vi "IMAQ Gerchberg Iteration.vi"(0 "field":T2, 1 "Original Source":dbl[][](array[numeric]), 2 "n_grid":i32=300, 3 "forward distance":dbl=0.02, 4 "Original Target":dbl[][](array[numeric]), 5 "error in (no error)":errorcluster, 6 "Source":T1, 7 "Target":T1, 8 "Source Phase":T1, 9 "Target Phase":T1) -> (10 "Source Intensity":dbl[][](array[numeric]), 11 "Target Intensity":dbl[][](array[numeric]), 12 "Source Phase":dbl[][](array[numeric]), 13 "Target Phase":dbl[][](array[numeric]), 14 "field out":T2, 15 "Target Intensity\n RMS Error":dbl(graph)=285.2404780234725, 19 "error out":errorcluster)   [LabVIEW 2012, in "LightPipes.lvlib"]
uses:
  LightPipes.lvlib
  <vilib>/vision/Image Controls.llb/IMAQ Image.ctl
panel:
  out "Source Phase":T1(plugin-control)
  out "Target Phase":T1(plugin-control)
  out "Source":T1(plugin-control)
  out "Target":T1(plugin-control)
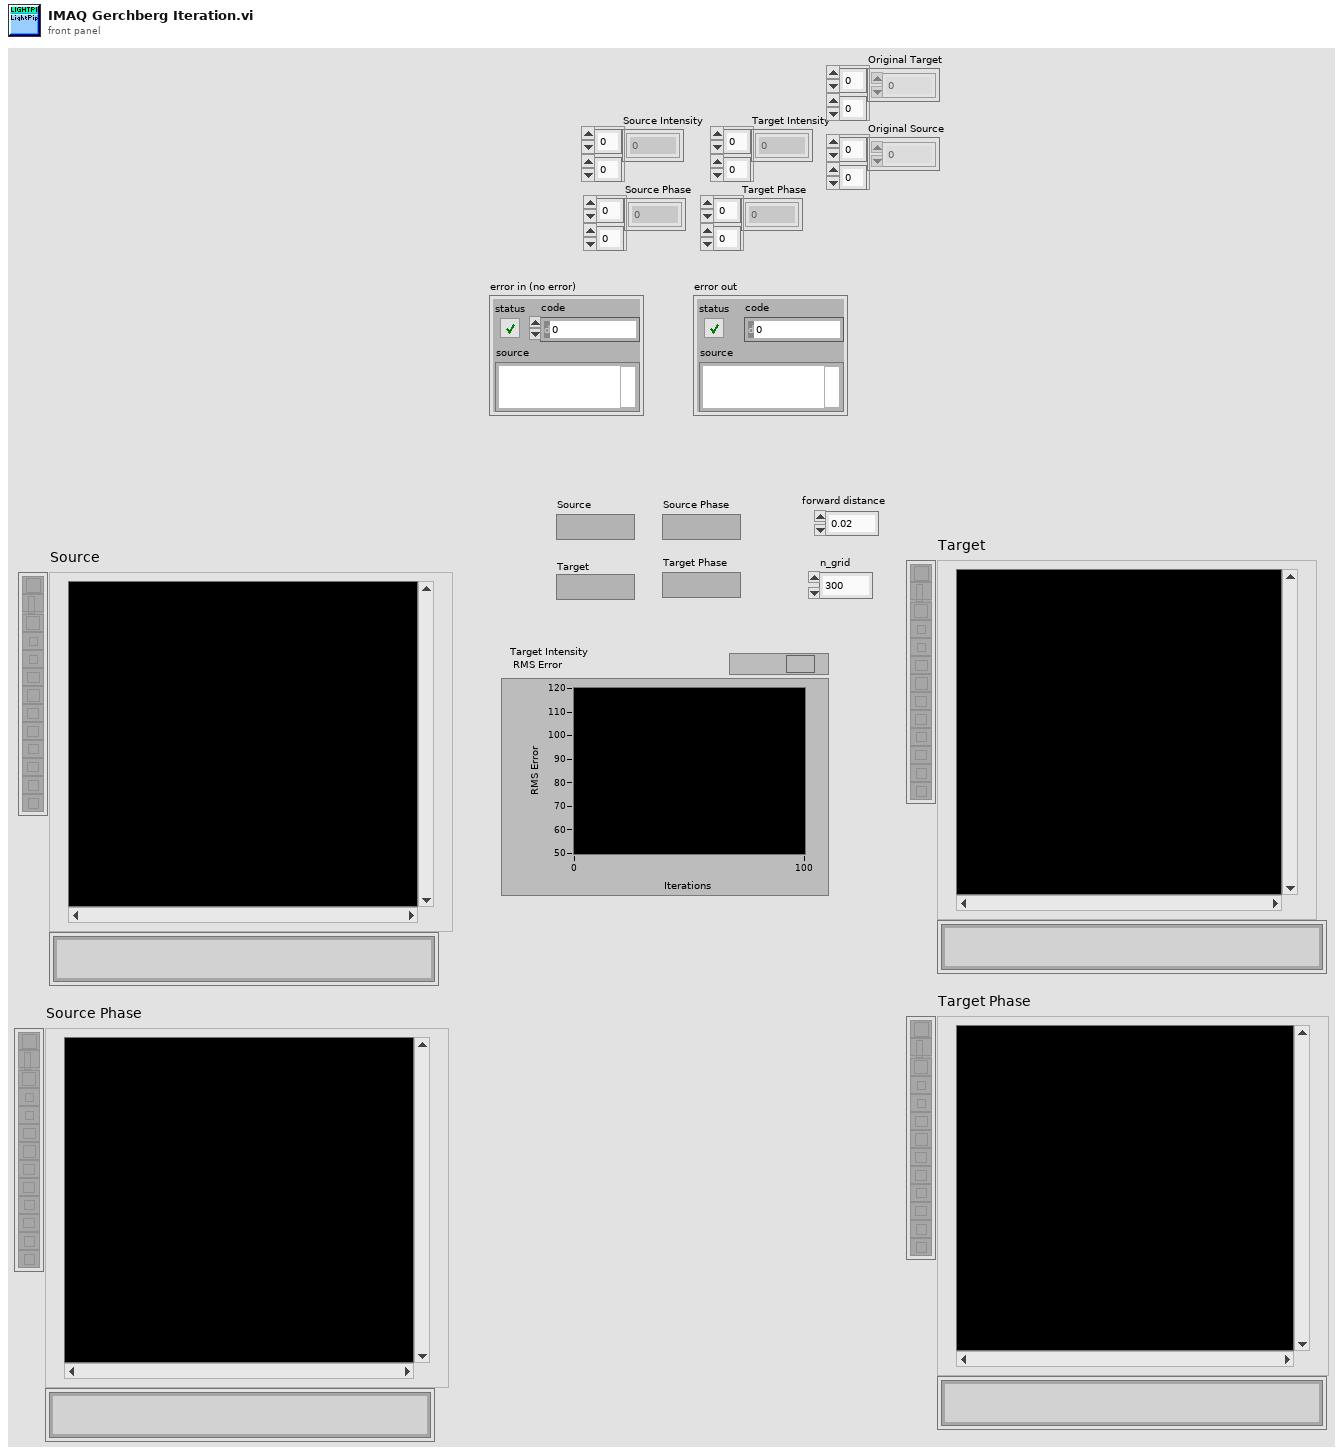
[diagram p1: front panel]
types:
  T1 = typedef "IMAQ Image.ctl" = refnum<image>
  T2 = cluster{"n_grid":i32, "@dummy control@":i8, "@dummy control@":i8, "@dummy control@":i8, "@dummy control@":i8, "size":dbl, "lambda":dbl, "int1":i32, "int2":i32, "int3":i32, "@dummy control@":i8, "@dummy control@":i8, "@dummy control@":i8, "@dummy control@":i8, "double1":dbl, "double2":dbl, "double3":dbl, "real":u32, "imaginary":u32}
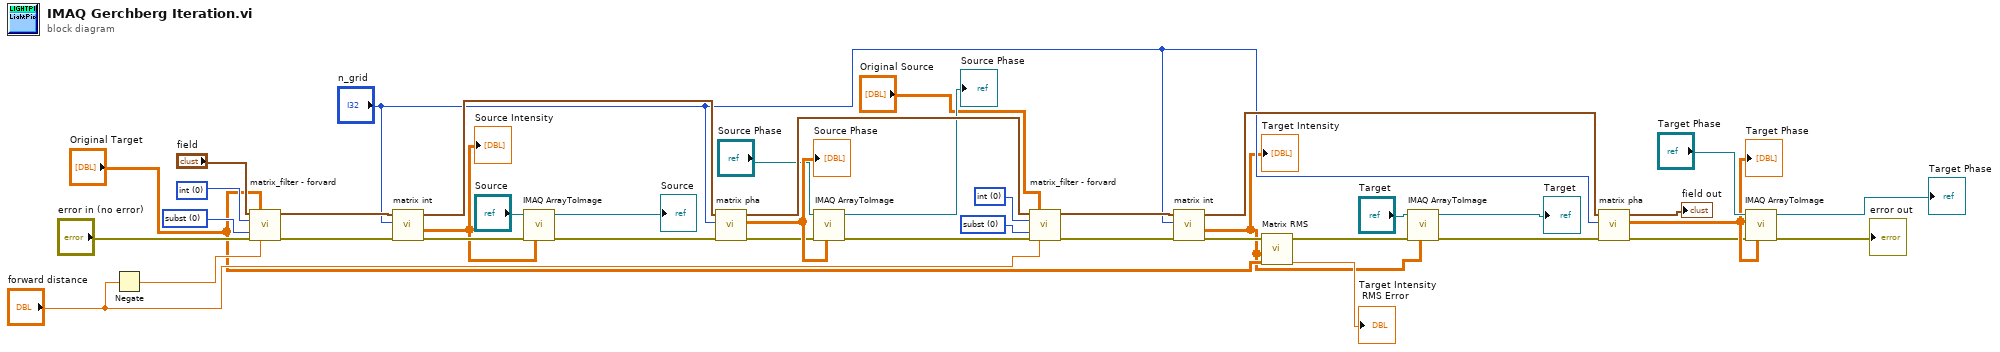
[diagram p0: block diagram]
diagram:
  w36 = i16 0 items=["int", "pha"] ("intensity/phase")
  w37 = i16 0 items=["subst", "mult"] ("multiplication/substitution")
  w38 = i16 0 items=["int", "pha"] ("intensity/phase")
  w39 = i16 0 items=["subst", "mult"] ("multiplication/substitution")
  n1 = Negate(x="forward distance") -> (-x=w35:dbl)
  n2 = call "matrix_filter - forvard.vi"("field"="field", "matrix in"="Original Target", "intensity/phase"=w36, "multiplication/substitution"=w37, "error in (no error)"="error in (no error)", "forward distance"=w35) -> ("field out"=w32:T2, "error out"=w23:errorcluster)  [unwired: 8 in]
  n3 = call "matrix int.vi"("error in (no error)"=w23, "n_grid"="n_grid", "field"=w32) -> ("error out"=w22:errorcluster, "matrix out 2D"=w3:dbl[][], "field out"=w31:T2)  [unwired: 6 in]
  "Source Intensity" <- w3
  n4 = call "IMAQ ArrayToImage"("Image Pixels (Float)"=w3, "error in (no error)"=w22, "Image"="Source") -> ("error out"=w21:errorcluster, "Image Out"=→"Source":T1)  [unwired: 7 in]
  n5 = call "matrix pha.vi"("error in (no error)"=w21, "n_grid"="n_grid", "field"=w31) -> ("error out"=w20:errorcluster, "matrix out 2D"=w28:dbl[][], "field out"=w30:T2)  [unwired: 6 in]
  "Source Phase" <- w28
  n6 = call "IMAQ ArrayToImage"("Image Pixels (Float)"=w28, "error in (no error)"=w20, "Image"="Source Phase") -> ("error out"=w19:errorcluster, "Image Out"=→"Source Phase":T1)  [unwired: 7 in]
  n7 = call "matrix_filter - forvard.vi"("field"=w30, "matrix in"="Original Source", "intensity/phase"=w38, "multiplication/substitution"=w39, "error in (no error)"=w19, "forward distance"="forward distance") -> ("field out"=w34:T2, "error out"=w18:errorcluster)  [unwired: 8 in]
  n8 = call "matrix int.vi"("error in (no error)"=w18, "n_grid"="n_grid", "field"=w34) -> ("error out"=w17:errorcluster, "matrix out 2D"=w1:dbl[][], "field out"=w33:T2)  [unwired: 6 in]
  "Target Intensity" <- w1
  n9 = call "Matrix RMS.vi"("Original Matrix"="Original Target", "Iterative Matrix"=w1, "error in (no error)"=w17) -> ("RMS"=→"Target Intensity\n RMS Error":dbl, "error out"=w16:errorcluster)  [unwired: 7 in]
  n10 = call "IMAQ ArrayToImage"("Image Pixels (Float)"=w1, "error in (no error)"=w16, "Image"="Target") -> ("error out"=w15:errorcluster, "Image Out"=→"Target":T1)  [unwired: 7 in]
  n11 = call "matrix pha.vi"("error in (no error)"=w15, "n_grid"="n_grid", "field"=w33) -> ("error out"=w14:errorcluster, "matrix out 2D"=w27:dbl[][], "field out"=→"field out":T2)  [unwired: 6 in]
  "Target Phase" <- w27
  n12 = call "IMAQ ArrayToImage"("Image Pixels (Float)"=w27, "error in (no error)"=w14, "Image"="Target Phase") -> ("error out"=→"error out":errorcluster, "Image Out"=→"Target Phase":T1)  [unwired: 7 in]
